vi "PH_Switch.ProcEvents.vi"(0 "i ref in":refnum<vi>, 5 "error in (no error)":errorcluster) -> (14 "i ref out":refnum<vi>, 19 "error out":errorcluster)   [LabVIEW 2014, in "PH_Switch.lvlib"]
doc: "This method is used to define the events the object will listen to. Add your own events here."
uses:
  PH_Switch.lvlib
  CSCore/BaseProcess/BaseProcess.event definition.ctl
  CSCore/CAEObj/CAEObj.event definition.ctl
  CSCore/BaseProcess/BaseProcess.descriptor string definition.ctl
  CSCore/BaseProcess/BaseProcess.lvlib
  CSCore/CAEObj/CAEObj.lvlib
  PH_Common/PH_Common.lvlib
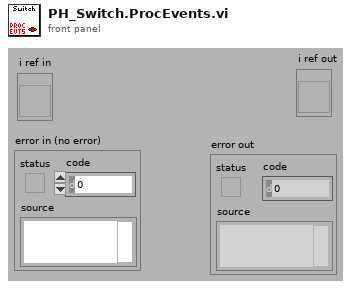
[diagram p1: front panel]
types:
  T1 = typedef "BaseProcess.lvlib/BaseProcess.event definition.ctl" = cluster{"CAEEvtDef":T2, "Data Descriptor":T3}
  T2 = typedef "CAEObj.lvlib/CAEObj.event definition.ctl" = cluster{"URL":string, "enable":bool, "ignoreResID":bool}
  T3 = typedef "BaseProcess.lvlib/BaseProcess.descriptor string definition.ctl" = string
  T4 = typedef "PH_Switch.lvlib/PH_Switch.i attribute.ctl" = cluster{"GUI Refs":T5, "Status true":T6, "Status false":T6, "Status Switch State":T6, "remote controlled":bool, "Tagname":cluster{"Switch":string, "True":string, "False":string}, "Beckhoff Instance":string, "Caption":cluster{"True":string, "False":string}, "Default State":string}
  T5 = typedef "PH_Switch.lvlib/PH_Switch.GUI Refs.ctl" = cluster{"true":refnum<vi>, "false":refnum<vi>, "Switch_state":refnum<vi>, "GUI-Knob":refnum<vi>, "Delete":refnum<vi>, "Function Textfield":refnum<vi>}
  T6 = typedef "PH_StatusHandler.lvlib/PH_StatusHandler.Status.ctl" = i16
  T7 = cluster{"Switch":string, "True":string, "False":string}
  T8 = typedef "PH_Common.lvlib/PH_DIM.Event Declarer.ctl" = cluster{"Service Name":string, "Selector":string}
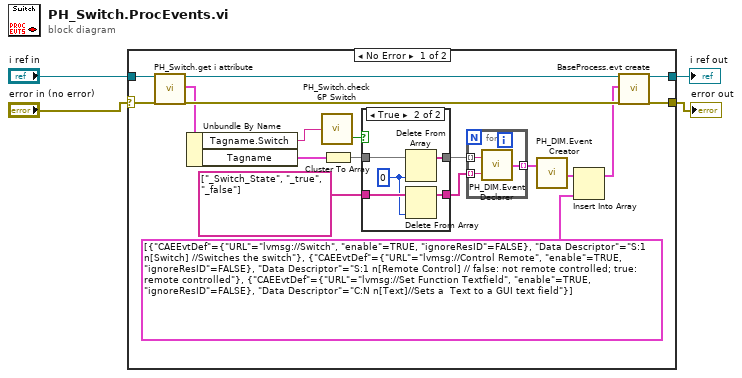
[diagram p0: block diagram]
diagram:
  n1 = case shown="No Error" "error in (no error)" {
    selector: "error in (no error)" -> [w16 w34]
    tunnel: "i ref in" -> [w5 w33]
    tunnel: [w21 w33] -> w3
    tunnel: [w20 w34] -> w2
    frame No Error {
      n2 = call "PH_Switch.get i attribute.vi"("i ref in"=w5, "error in (no error)"=w16) -> ("i ref out"=w10:refnum<vi>, "i attribute"=w9:T4, "error out"=w22:errorcluster)  [unwired: 15 in]
      n3 = Unbundle By Name(w9) -> ("Tagname.Switch"=w6:string, "Tagname"=w8:T7)
      n4 = call "PH_Switch.check 6P Switch.vi"("Tagname"=w6) -> ("6P Switch?"=w11:bool)  [unwired: 1 out]
      n5 = Cluster To Array(cluster=w8) -> (array=w7:string[])
      n6 = case shown="True" w11 {
        tunnel: w7 -> [w24 w29]
        tunnel: [w24 w28] -> w14
        tunnel: string[] ["_Switch_State", "_true", "_false"] -> [w23 w27]
        tunnel: [w23 w26] -> w12
        frame False {
        }
        frame True {
          w25 = 0 ("index")
          n7 = Delete From Array(array=w29, index=w25) -> (array with subset deleted=w28:string[])  [unwired: 1 in, 1 out]
          n8 = Delete From Array(array=w27, index=w25) -> (array with subset deleted=w26:string[])  [unwired: 1 in, 1 out]
        }
      }
      n9 = for {
        tunnel: [w32] -> w18 mode=indexing
        tunnel: w14 -> [w31] mode=indexing
        tunnel: w12 -> [w30] mode=indexing
        n10 = call "PH_DIM.Event Declarer.vi"("Selector"=w30, "Service Name"=w31) -> ("declared DIM Event"=w32:T8)
      }
      n11 = call "PH_DIM.Event Creator.vi"("Trendmessage Services"=w18) -> ("DIM Service Events"=w19:T1[])  [unwired: 18 in]
      n12 = Insert Into Array(array=w19, new element=T1[] [{"CAEEvtDef"={"URL"="lvmsg://Switch", "enable"=TRUE, "ignoreResID"=FALSE}, "Data Descriptor"="S:1 n[Switch] //Switches the switch"}, {"CAEEvtDef"={"URL"="lvmsg://Control Remote", "enable"=TRUE, "ignoreResID"=FALSE}, "Data Descriptor"="S:1 n[Remote Control] // false: not remote controlled; true: remote controlled"}, {"CAEEvtDef"={"URL"="lvmsg://Set Function Textfield", "enable"=TRUE, "ignoreResID"=FALSE}, "Data Descriptor"="C:N n[Text]//Sets a  Text to a GUI text field"}] ("new events")) -> (w17:T1[])  [unwired: 1 in]
      n13 = call "BaseProcess.evt create.vi"("i ref in"=w10, "newEvents"=w17, "error in (no error)"=w22) -> ("i ref out"=w21:refnum<vi>, "error out"=w20:errorcluster)  [unwired: 13 in, 2 out]
    }
    frame Error {
    }
  }
  "i ref out" <- w3
  "error out" <- w2
